vi "Runtime Test.vi"() -> ()   [LabVIEW 2014, in "io plugin tests.lvlib"]
doc: "This VI shows an example for how to test the Runtime functionality of the module. This will need to be modified according to module functionality."
uses:
  io plugin tests.lvlib
  module/execution/tag bus configurable plugin module.lvclass
  <vilib>/NI/Tag Bus/dictionary/data dictionary.lvclass/data dictionary.ctl
  <vilib>/NI/Tag Bus/dictionary/lookup polymorphs/locate double.vi
  <vilib>/NI/Tag Bus/table/data polymorphs/read one/read Double.vi
  <vilib>/NI/Tag Bus/table/data polymorphs/write one/write Double.vi
  <vilib>/NI/Tag Bus/dictionary/search/find data index.vi
  <vilib>/NI/Tag Bus/dictionary/search/search string list.vi
  <vilib>/NI/Tag Bus/dictionary/tag not found.vi
  module/configuration/tag bus configurable plugin module configuration.lvclass
  <vilib>/NI/Tag Bus/dictionary/data dictionary.lvclass
  <vilib>/NI/Tag Bus/table/data table.lvlib
panel:
  out "Input":dbl
  out "Processing Result":dbl
  in  "Processing Parameters":dbl
  in  "output value":dbl=42.0 format="%#_13g"
  out "error":errorcluster
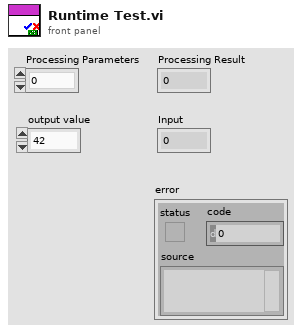
[diagram p1: front panel]
types:
  T1 = typedef "TBM channel.lvclass/data tables.ctl" = cluster{"input data":T2, "processing parameter":T2, "processing result":T2, "output data":T2}
  T2 = typedef "tag bus.lvlib/dictionary table pair.ctl" = cluster{"data dictionary":refnum<class "data dictionary.lvclass">, "data table":T3}
  T3 = typedef "tag bus.lvlib/data table.lvlib/data table.ctl" = cluster{"Double":dbl[], "Single":sgl[], "I64":i64[], "I32":i32[], "I16":i16[], "I8":i8[], "U64":u64[], "U32":u32[], "U16":u16[], "U8":u8[], "Boolean":bool[], "String":string[], "Array of Double":cluster{"DBL Array":dbl[]}[], "Array of Single":cluster{"SGL Array":sgl[]}[], "Array of I64":cluster{"I64 Array":i64[]}[], "Array of I32":cluster{"I32 Array":i32[]}[], "Array of I16":cluster{"I16 Array":i16[]}[], "Array of I8":cluster{"I8 Array":i8[]}[], "Array of U64":cluster{"U64 Array":u64[]}[], "Array of U32":cluster{"U32 Array":u32[]}[], "Array of U16":cluster{"U16 Array":u16[]}[], "Array of U8":cluster{"U8 Array":u8[]}[], "Array of Boolean":cluster{"Boolean Array":bool[]}[], "Array of String":cluster{"String Array":string[]}[]}
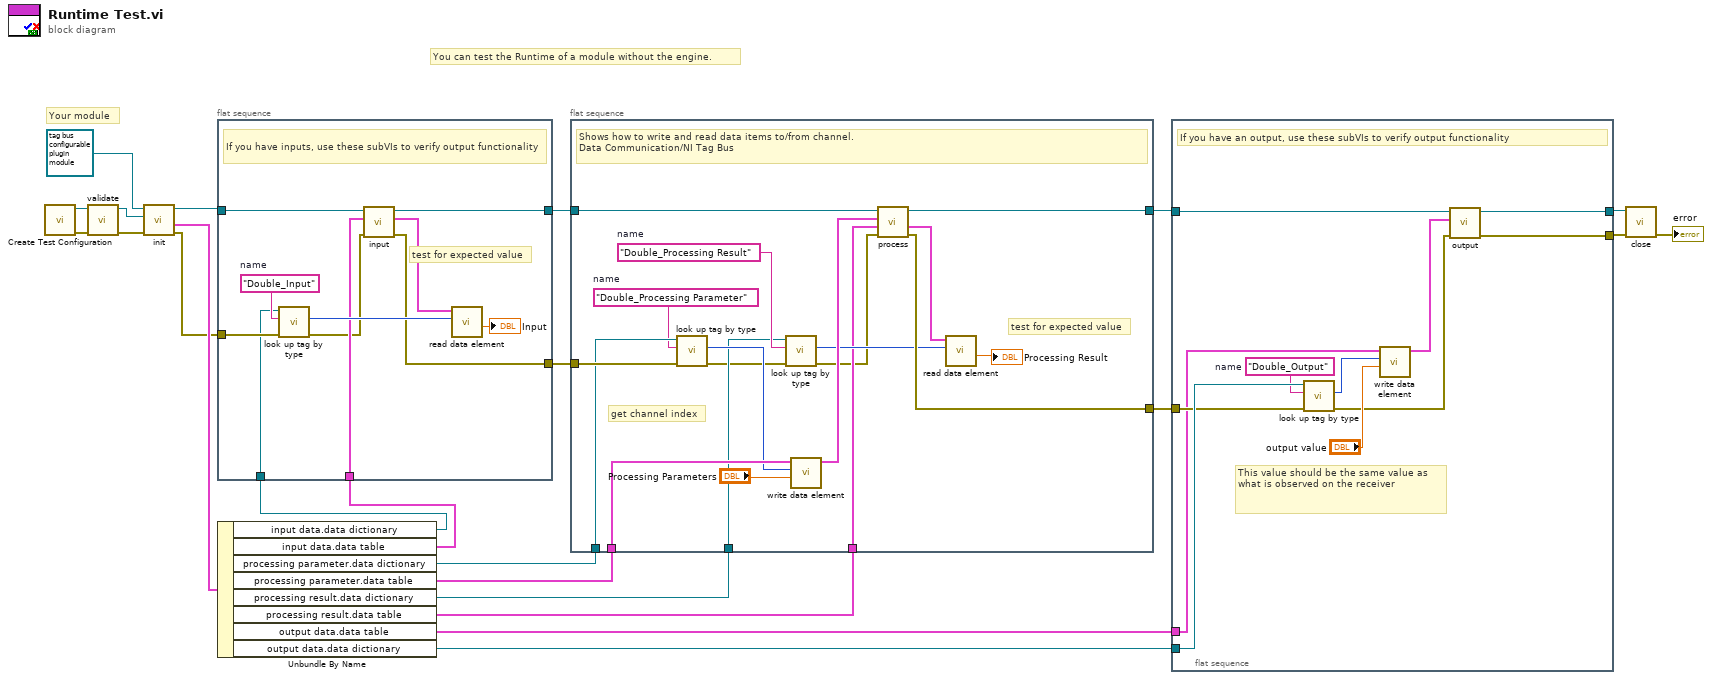
[diagram p0: block diagram]
diagram:
  # "You can test the Runtime of a module without the engine."
  # "Your module"
  n1 = call "Create Test Configuration.vi"() -> ("error out"=w19:errorcluster, "Module Configuration"=w20:refnum<class "tag bus configurable plugin module configuration.lvclass">)  [unwired: 6 in, 4 out]
  n2 = call-dynamic "validate.vi"("error in"=w19, "tag bus configurable plugin module configuration in"=w20) -> ("error out"=w22:errorcluster, "tag bus configurable plugin module configuration out"=w21:refnum<class "tag bus configurable plugin module configuration.lvclass">)  [unwired: 8 in]
  n3 = call-dynamic "init.vi"("error in"=w22, "TBM module configuration in"=w21, "tag bus configurable plugin module in"=refnum<class "tag bus configurable plugin module.lvclass"> refnum ("tag bus configurable plugin module")) -> ("error out"=w1:errorcluster, "data allocations"=w2:T1, "tag bus configurable plugin module out"=w3:refnum<class "tag bus configurable plugin module.lvclass">)  [unwired: 5 in, 1 out]
  n4 = flat-sequence {
    tunnel: w1 -> [w31]
    tunnel: [w26] -> w9
    tunnel: w3 -> [w34]
    tunnel: [w33] -> w8
    tunnel: w7 -> [w30]
    tunnel: w4 -> [w27]
    frame #0 {
      w32 = "Double_Input"  # name
      # "test for expected value"
      # "If you have inputs, use these subVIs to verify output functionality"
      n5 = call-poly <vilib>:"look up tag by type.vi"("error in"=w31, "name"=w32, "data dictionary in"=w30) -> ("error out"=w25:errorcluster, "index"=w28:i32)  [unwired: 6 in, 1 out]
      n6 = call-dynamic "input.vi"("error in"=w25, "data table in"=w27, "tag bus configurable plugin module in"=w34) -> ("error out"=w26:errorcluster, "data table out"=w29:T3, "tag bus configurable plugin module out"=w33:refnum<class "tag bus configurable plugin module.lvclass">)  [unwired: 6 in]
      n7 = call-poly <vilib>:"read data element.vi"("index"=w28, "data table in"=w29) -> ("value"=→"Input":dbl)  [unwired: 8 in, 1 out]
    }
  }
  n8 = Unbundle By Name(w2) -> ("input data.data dictionary"=w7:refnum<class "data dictionary.lvclass">, "input data.data table"=w4:T3, "processing parameter.data dictionary"=w18:refnum<class "data dictionary.lvclass">, "processing parameter.data table"=w17:T3, "processing result.data dictionary"=w6:refnum<class "data dictionary.lvclass">, "processing result.data table"=w5:T3, "output data.data table"=w10:T3, "output data.data dictionary"=w16:refnum<class "data dictionary.lvclass">)
  n9 = flat-sequence {
    tunnel: w18 -> [w43]
    tunnel: w9 -> [w44]
    tunnel: w17 -> [w52]
    tunnel: [w51] -> w12
    tunnel: [w50] -> w11
    tunnel: w8 -> [w48]
    tunnel: w6 -> [w41]
    tunnel: w5 -> [w39]
    frame #0 {
      w42 = "Double_Processing Parameter"  # name
      w46 = "Double_Processing Result"  # name
      # "test for expected value"
      # "get channel index"
      # "Shows how to write and read data items to/from channel.\nData Communication/NI Tag Bus"
      n10 = call-poly <vilib>:"look up tag by type.vi"("error in"=w44, "name"=w42, "data dictionary in"=w43) -> ("error out"=w38:errorcluster, "index"=w45:i32)  [unwired: 6 in, 1 out]
      n11 = call-poly <vilib>:"look up tag by type.vi"("error in"=w38, "name"=w46, "data dictionary in"=w41) -> ("error out"=w37:errorcluster, "index"=w47:i32)  [unwired: 6 in, 1 out]
      n12 = call-poly <vilib>:"write data element.vi"("value"="Processing Parameters", "index"=w45, "data table in"=w52) -> ("data table out"=w49:T3)  [unwired: 8 in]
      n13 = call-dynamic "process.vi"("error in"=w37, "result allocation"=w39, "parameters"=w49, "module in"=w48) -> ("error out"=w50:errorcluster, "results"=w40:T3, "module out"=w51:refnum<class "tag bus configurable plugin module.lvclass">)  [unwired: 4 in, 1 out]
      n14 = call-poly <vilib>:"read data element.vi"("index"=w47, "data table in"=w40) -> ("value"=→"Processing Result":dbl)  [unwired: 8 in, 1 out]
    }
  }
  n15 = flat-sequence {
    tunnel: w16 -> [w63]
    tunnel: [w59] -> w15
    tunnel: [w58] -> w14
    tunnel: w12 -> [w57]
    tunnel: w11 -> [w56]
    tunnel: w10 -> [w55]
    frame #0 {
      w53 = "Double_Output"  # name
      # "This value should be the same value as what is observed on the receiver"
      # "If you have an output, use these subVIs to verify output functionality"
      n16 = call-poly <vilib>:"look up tag by type.vi"("error in"=w56, "name"=w53, "data dictionary in"=w63) -> ("error out"=w54:errorcluster, "index"=w62:i32)  [unwired: 6 in, 1 out]
      n17 = call-poly <vilib>:"write data element.vi"("value"="output value", "index"=w62, "data table in"=w55) -> ("data table out"=w60:T3)  [unwired: 8 in]
      n18 = call-dynamic "output.vi"("error in"=w54, "data table in"=w60, "tag bus configurable plugin module in"=w57) -> ("error out"=w58:errorcluster, "tag bus configurable plugin module out"=w59:refnum<class "tag bus configurable plugin module.lvclass">)  [unwired: 6 in, 1 out]
    }
  }
  n19 = call-dynamic "close.vi"("error in"=w14, "tag bus configurable plugin module in"=w15) -> ("error out"=→"error":errorcluster)  [unwired: 9 in]
